vi "match-string.vi"(9 "match string":string="2334", 11 "String":string="wwewewewew2334fgfgdfs") -> (3 "match?(True=match)":bool)   [LabVIEW 2011]
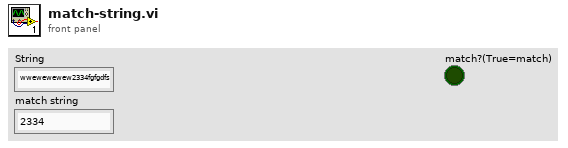
[diagram p1: front panel]
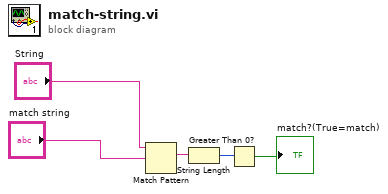
[diagram p0: block diagram]
diagram:
  n1 = Match Pattern(string="String", regular expression="match string") -> (match substring=w2:string)  [unwired: 1 in, 3 out]
  n2 = String Length(string=w2) -> (length=w3:i32)
  n3 = Greater Than 0?(x=w3) -> (x > 0?=→"match?(True=match)":bool)
